vi "WRITE SINGLE FUN.vi"(8 "error in (no error)":errorcluster, 10 "data":dbl[](array[numeric]), 11 "XNET Signal":refnum<k21>="IsolationStatus\nEDriveMfile_20230607") -> (0 "error out":errorcluster, 2 "session out 2":refnum<k21>)   [LabVIEW 2018]
uses:
  <vilib>/xnet/xnet.llb/XNET Create Session (Signal Output Single-point).vi
  <vilib>/xnet/xnet.llb/XNET Write (Signal Single-point).vi
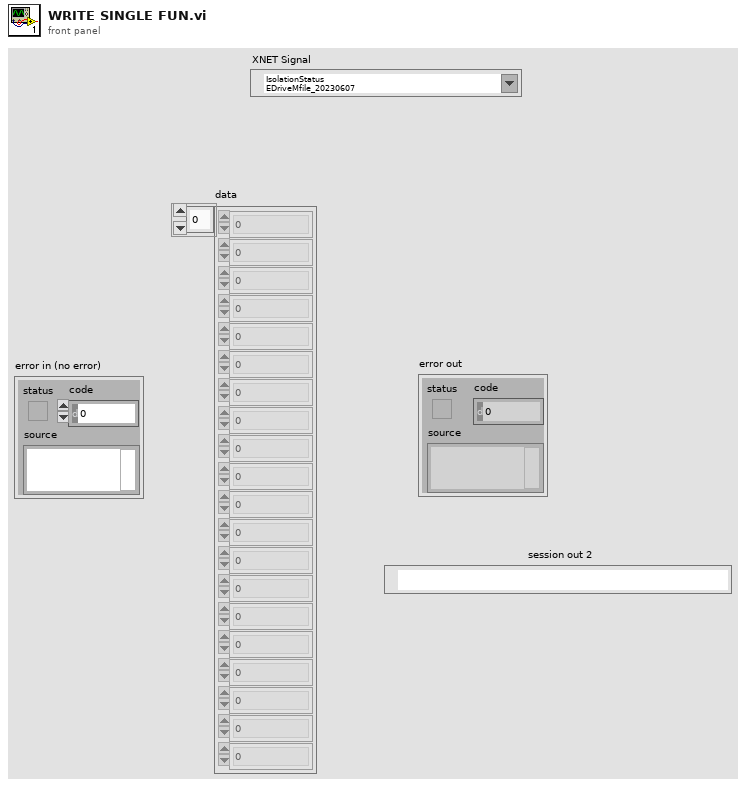
[diagram p1: front panel]
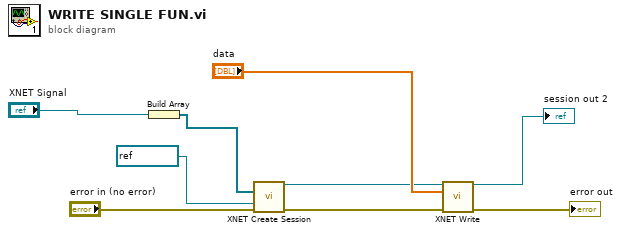
[diagram p0: block diagram]
diagram:
  n1 = Build Array("XNET Signal") -> (w3:refnum<k21>[])
  n2 = call-poly <vilib>:"XNET Create Session.vi"("signal list"=w3, "interface"=refnum<k21> "CAN1" ("Select Interface"), "error in (no error)"="error in (no error)") -> ("session out"=w5:refnum<k21>, "error out"=w4:errorcluster)  [unwired: 11 out]
  n3 = call-poly <vilib>:"XNET Write.vi"("session in"=w5, "data"="data", "error in (no error)"=w4) -> ("session out"=→"session out 2":refnum<k21>, "error out"=→"error out":errorcluster)  [unwired: 11 in]
